vi "Set Argument - Arguments Array.vi"(7 "Function Name":string, 8 "Error In":errorcluster, 9 "Args Array":string[][](array[string]), 11 "OPI Ref":refnum<data-value>) -> (0 "Error Out":errorcluster, 3 "OPI Ref":refnum<data-value>)   [LabVIEW 2020, in "OPI.lvclass"]
doc: "Set all arguments values for the future function specified by Function Name. \n\nThe wired 2D array should represent the pairs of argument name and pythonic value. This array can be obtained by Get Arguments method. This way multiple sets of values for arguments can be stored and re-applied at any time, before the function call.\n\nThe values are transmitted to the PES. This optimizes the speed with which calls can be made, because no data needs to be transmitted at call time."
uses:
  OPI.lvclass
  OPI.lvclass/OPI.ctl
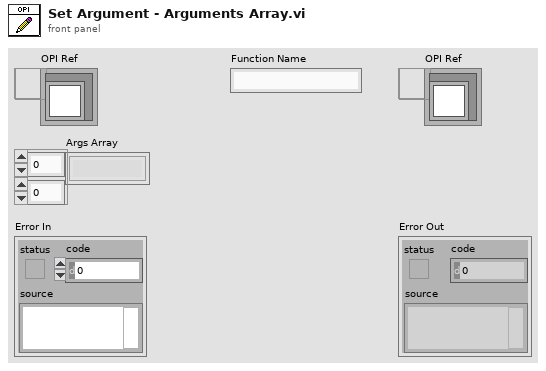
[diagram p1: front panel]
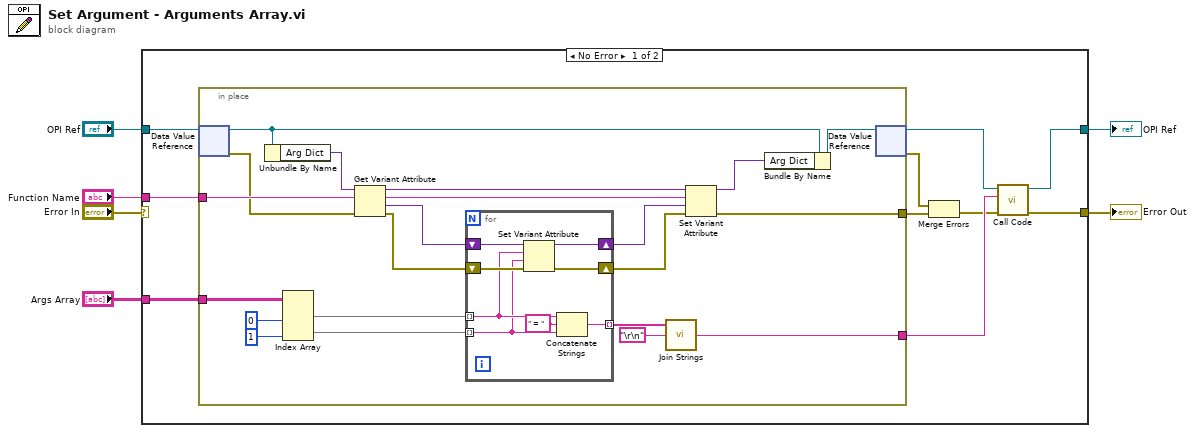
[diagram p0: block diagram]
diagram:
  n1 = case shown="No Error" "Error In" {
    selector: "Error In" -> [_ w45]
    tunnel: "OPI Ref" -> [w16 w46]
    tunnel: "Function Name" -> [w15 _]
    tunnel: [w13 w46] -> w4
    tunnel: "Args Array" -> [w12 _]
    tunnel: [w7 w45] -> w1
    frame No Error {
      n2 = in-place {
        in-place-border: w15 -> [w32]
        in-place-border: w12 -> [w24]
        in-place-border: [w17] -> w11
        in-place-border: [w25] -> w10
        n3 = in-place-dvr #1(w16) -> (w31:refnum<class "OPI.lvclass">, w28:errorcluster)
        n4 = Unbundle By Name(w31) -> ("Arg Dict"=w36:variant)
        n5 = Index Array(array=w24, index (col) #1=0 ("disabled index (col)"), index (col) #2=1 ("index (col)")) -> (element #1=w21:string[], element #2=w20:string[])  [unwired: 2 in]
        n6 = Get Variant Attribute(Variant=w36, name=w32, error in=w28) -> (duplicate Variant=w34:variant, value=w35:variant, error out=w27:errorcluster)  [unwired: 1 in, 1 out]
        n7 = for {
          shift-right: [w43] -> w33
          shift-left: w35 -> [w44]
          shift-right: [w41] -> w26
          shift-left: w27 -> [w42]
          tunnel: w21 -> [w39] mode=indexing
          tunnel: w20 -> [w38] mode=indexing
          tunnel: [w37] -> w19 mode=indexing
          n8 = Set Variant Attribute(Variant=w44, name=w39, value=w38, error in=w42) -> (Variant out=w43:variant, error out=w41:errorcluster)  [unwired: 1 out]
          n9 = Concatenate Strings(w39, " = " ("string"), w38) -> (w37:string)
        }
        n10 = call <vilib>:"Join Strings.vi"("Separator (,)"="\r\n", "Strings In"=w19) -> ("String"=w17:string)  [unwired: 1 in]
        n11 = Set Variant Attribute(Variant=w34, name=w32, value=w33, error in=w26) -> (Variant out=w30:variant, error out=w25:errorcluster)  [unwired: 1 out]
        n12 = Bundle By Name(cluster=w31, "Arg Dict"=w30) -> (w29:refnum<class "OPI.lvclass">)
        n13 = in-place-dvr #1(w29) -> (w14:refnum<data-value>, w9:errorcluster)
      }
      n14 = Merge Errors(w9, w10) -> (w8:errorcluster)
      n15 = call "Call Code.vi"("Error In"=w8, "Pythonic Code"=w11, "OPI Ref"=w14) -> ("Error Out"=w7:errorcluster, "OPI Ref"=w13:refnum<data-value>)  [unwired: 7 in]
    }
    frame Error {
    }
  }
  "Error Out" <- w1
  "OPI Ref" <- w4
